vi "openDocuement.vi"(8 "error in (no error)":errorcluster, 11 "MS-Word in":refnum<class "MS-Word.lvclass">) -> (0 "error out":errorcluster, 3 "MS-Word out":refnum<class "MS-Word.lvclass">)   [LabVIEW 2017, in "LabVIEW NPOI.lvlib" / "MS-Word.lvclass"]
doc: "Protected dynamic dispatch method to open the <b>Document</b> file located at <b>File Path</b> for reading."
uses:
  MS-Word.lvclass
  C:/Users/Neo/Desktop/Dev_Tools_BR/LabVIEW_NPOI/src/LabVIEW NPOI/Document/Document.lvclass
  Document/Document.lvclass/Document.ctl
  MS-Word.lvclass/MS-Word.ctl
  Document/Get FilePath.vi
  xwpfWriter/xwpfWriter.lvclass
  xwpfReader/xwpfReader.lvclass
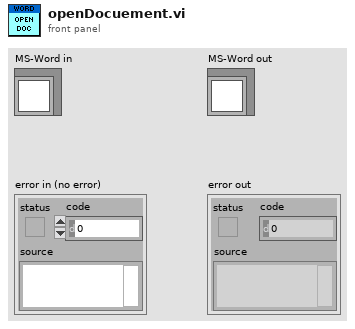
[diagram p1: front panel]
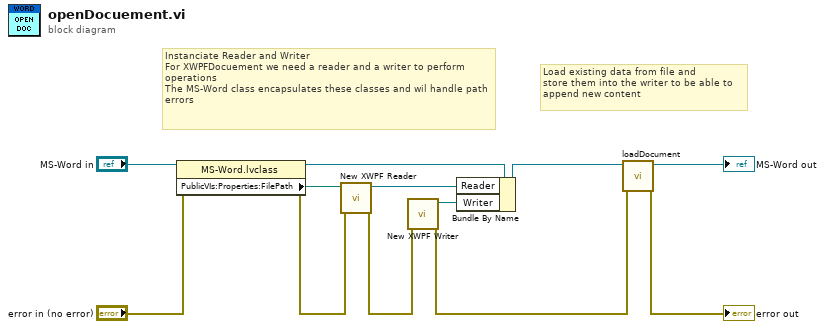
[diagram p0: block diagram]
diagram:
  # "Load existing data from file and\nstore them into the writer to be able to\nappend new content"
  # "Instanciate Reader and Writer\nFor XWPFDocuement we need a reader and a writer to perform operations\nThe MS-Word class encapsulates these classes and wil handle path errors"
  n1 = property class="MS-Word.lvclass"(reference="MS-Word in", error in="error in (no error)") -> (reference out=w9:refnum<class "MS-Word.lvclass">, error out=w6:errorcluster, "PublicVIs:Properties:FilePath"=w10:path)
  n2 = call "New XWPF Reader.vi"("error in (no error)"=w6, "XWPF File Path"=w10) -> ("error out"=w5:errorcluster, "xwpfReader out"=w8:refnum<class "xwpfReader.lvclass">)  [unwired: 8 in]
  n3 = call "New XWPF Writer.vi"("error in (no error)"=w5) -> ("error out"=w2:errorcluster, "xwpfWriter out"=w7:refnum<class "xwpfWriter.lvclass">)  [unwired: 9 in]
  n4 = Bundle By Name(cluster=w9, "Reader"=w8, "Writer"=w7) -> (w4:refnum<class "MS-Word.lvclass">)
  n5 = call "loadDocument.vi"("error in (no error)"=w2, "MS-Word in"=w4) -> ("error out"=→"error out":errorcluster, "MS-Word out"=→"MS-Word out":refnum<class "MS-Word.lvclass">)  [unwired: 8 in]
